vi "Query.vi"(8 "error in (no error)":errorcluster, 9 "current time":timestamp, 10 "gRPCid":T1) -> (0 "error out":errorcluster)   [LabVIEW 2019, in "ctet_smu User Library.lvlib"]
uses:
  ctet_smu User Library.lvlib
  Servers/ctet_smu/gRPC lvSupport/Server API/typeDefs/grpcId.ctl
  Servers/ctet_smu/ctet_smu Class/RPC Messages/measurementservice_QueryResponse/measurementservice_QueryResponse_Data.ctl
  Servers/ctet_smu/ctet_smu Class/ctet_smu.lvclass
  Servers/ctet_smu/gRPC lvSupport/gprc-lvsupport.lvlib
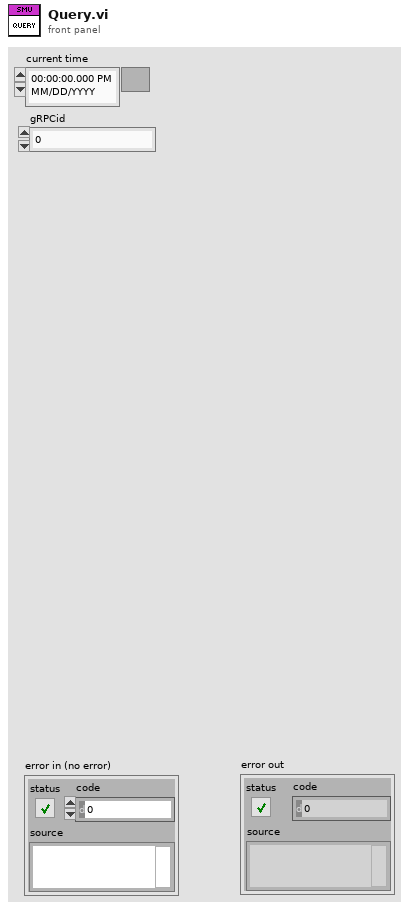
[diagram p1: front panel]
types:
  T1 = typedef "ctet_smu.lvlib/gprc-lvsupport.lvlib/grpcId.ctl" = u64
  T2 = typedef "ctet_smu.lvlib/ctet_smu.lvclass/measurementservice_QueryResponse_Data.ctl" = cluster{"message":string, "status":i64}
  T3 = typedef "ctet_smu.lvlib/ctet_smu.lvclass/measurementservice_QueryRequest_Data.ctl" = cluster{"query":string}
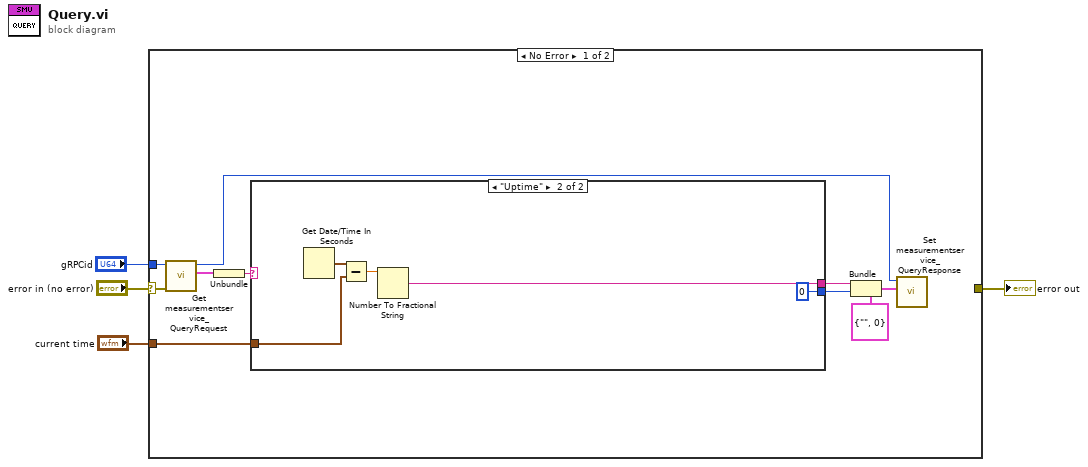
[diagram p0: block diagram]
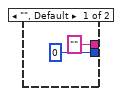
[diagram p2: hidden frame]
diagram:
  n1 = case shown="No Error" "error in (no error)" {
    selector: "error in (no error)" -> [w9 w22]
    tunnel: [_ w22] -> w4
    tunnel: "current time" -> [w13 _]
    tunnel: "gRPCid" -> [w10 _]
    frame No Error {
      n2 = call "Get measurementservice_QueryRequest.vi"("error in (no error)"=w9, "gRPCid"=w10) -> ("Message Data"=w8:T3, "gRPCid out"=w7:T1)  [unwired: 7 in, 1 out]
      n3 = Unbundle(w8) -> ("query"=w14:string)
      n4 = case shown="\"Uptime\"" w14 {
        tunnel: w13 -> [_ w20]
        tunnel: ["" w18] -> w12
        tunnel: [i64 0 ("status") i64 0 ("status")] -> w11
        frame "", Default {
        }
        frame "Uptime" {
          n5 = Get Date/Time In Seconds() -> (seconds since 1Jan1904=w21:timestamp)
          n6 = Subtract(x=w21, y=w20) -> (x-y=w19:dbl)
          n7 = Number To Fractional String(number=w19) -> (F-format string=w18:string)  [unwired: 3 in]
        }
      }
      n8 = Bundle(cluster=T2 {"message"="", "status"=0} ("Message Data"), "message"=w12, "status"=w11) -> (w5:T2)
      n9 = call "Set measurementservice_QueryResponse.vi"("Message Data"=w5, "gRPCid"=w7) -> ()  [unwired: 9 in, 1 out]
    }
    frame Error {
    }
  }
  "error out" <- w4
